vi "Enqueue Message (Single).vi"(6 "Priority Message? (F)":bool, 8 "error in (no error)":errorcluster, 9 "Message Data":variant, 10 "Message":string, 11 "Message Queue":refnum<queue>) -> (0 "error out":errorcluster, 3 "dup Message Queue":refnum<queue>)   [LabVIEW 2017, in "Message Queue.lvlib"]
doc: "For a regular message, enqueue the message. For a priority message, enqueue it at the front of the queue."
uses:
  Message Queue.lvlib
  Message Cluster.ctl
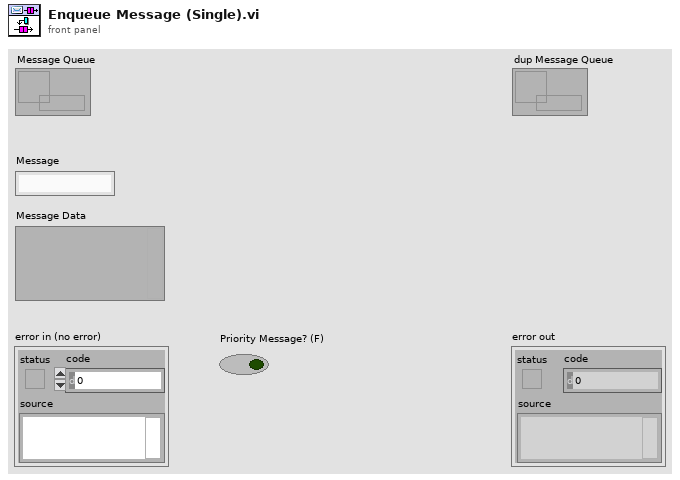
[diagram p1: front panel]
types:
  T1 = typedef "Message Queue.lvlib/Message Cluster.ctl" = cluster{"Message":string, "Message Data":variant}
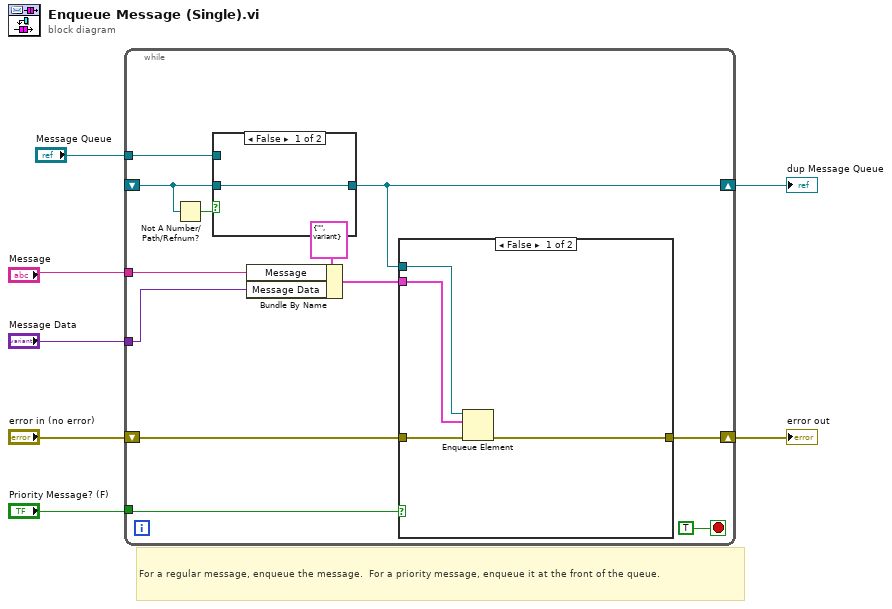
[diagram p0: block diagram]
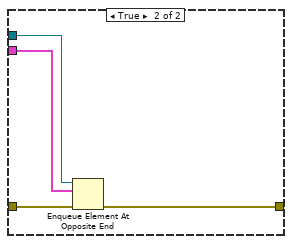
[diagram p3: hidden frame]
diagram:
  # "For a regular message, enqueue the message.  For a priority message, enqueue it at the front of the queue."
  n1 = while {
    tunnel: "Message" -> [w18]
    tunnel: "Message Data" -> [w17]
    tunnel: "Priority Message? (F)" -> [w16]
    shift-right: [w14] -> w3
    shift-left: "error in (no error)" -> [w15]
    shift-right: [w10] -> w2
    shift-left: _ -> [w9]
    tunnel: "Message Queue" -> [w8]
    stop <- TRUE stop-if-true
    n2 = Not A Number/Path/Refnum?(number/path/refnum=w9) -> (NaN/Path/Refnum?=w11:bool)
    n3 = case shown="False" w11 {
      tunnel: [w20 w21] -> w10
      tunnel: w9 -> [w20 _]
      tunnel: w8 -> [_ w21]
      frame False {
      }
      frame True {
      }
    }
    n4 = Bundle By Name(cluster=T1 {"Message"="", "Message Data"=variant} ("Message Cluster"), "Message"=w18, "Message Data"=w17) -> (w13:T1)
    n5 = case shown="False" w16 {
      tunnel: w15 -> [w25 w29]
      tunnel: [w24 w28] -> w14
      tunnel: w10 -> [w23 w27]
      tunnel: w13 -> [w22 w26]
      frame False {
        n6 = Enqueue Element(queue=w23, element=w22, error in (no error)=w25) -> (error out=w24:errorcluster)  [unwired: 1 in, 2 out]
      }
      frame True {
        n7 = Enqueue Element At Opposite End(queue=w27, element=w26, error in (no error)=w29) -> (error out=w28:errorcluster)  [unwired: 1 in, 2 out]
      }
    }
  }
  "error out" <- w3
  "dup Message Queue" <- w2
